vi "calculate alpha.vi"(7 "Substance (CO2/H2O)":T1, 8 "P [kPa]":dbl format="%#_13g", 9 "T [K]":dbl, 10 "Psi_i":dbl, 11 "Chi_i":dbl) -> (3 "absorptance_i":dbl)   [LabVIEW 2017, in "LicorLI7000.lvlib"]
uses:
  LicorLI7000.lvlib
  conventions/Substance.ctl
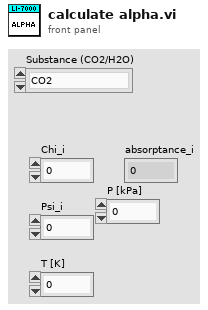
[diagram p1: front panel]
types:
  T1 = typedef "LicorLI7000.lvlib/Substance.ctl" = enum16{"CO2", "H2O"}
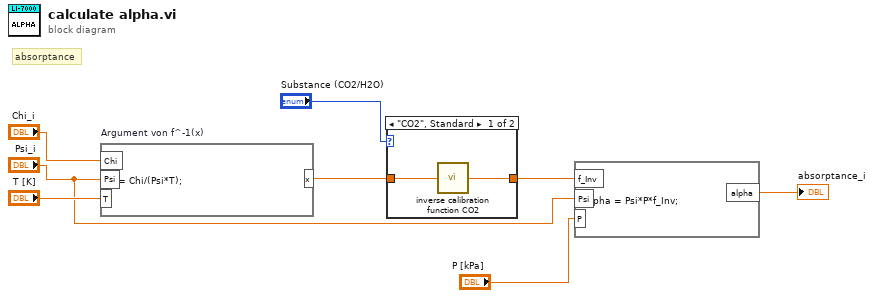
[diagram p0: block diagram]
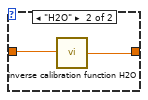
[diagram p2: hidden frame]
diagram:
  # "absorptance"
  n1 = formula code="x = Chi/(Psi*T);" "Argument von f^-1(x)"("Chi"="Chi_i", "Psi"="Psi_i", "T"="T [K]") -> ("x"=w8:dbl)
  n2 = case shown="\"CO2\", Standard" "Substance (CO2/H2O)" {
    tunnel: w8 -> [w10 w12]
    tunnel: [w9 w11] -> w5
    frame "CO2", Default {
      n3 = call "inverse calibration function CO2.vi"("x"=w10) -> ("f_inv(x)"=w9:dbl)  [unwired: 14 in]
    }
    frame "H2O" {
      n4 = call "inverse calibration function H2O.vi"("x"=w12) -> ("f_inv(x)"=w11:dbl)  [unwired: 14 in]
    }
  }
  n5 = formula code="alpha = Psi*P*f_Inv;"("f_Inv"=w5, "Psi"="Psi_i", "P"="P [kPa]") -> ("alpha"=→"absorptance_i":dbl)
